vi "test Data Width and Data Loss Error (Integer).vi"(8 "error in (no error)":errorcluster, 11 "TestCase in":refnum<class "BCD.lvclass">) -> (0 "error out":errorcluster, 3 "TestCase out":refnum<class "BCD.lvclass">)   [LabVIEW 2027, in "BCD.lvclass"]
uses:
  BCD.lvclass
  89223b31-db80-4792-afa8-2a57f7cc7b8f.vi
  a83072f1-e87d-421c-9031-0ad09725bb69.vi
  eb97fcc3-29ee-467e-b675-3d761fb83be5.vi
  24b16479-40f3-4730-80e6-3775a7937614.vi
  Source/Get Bits Per Digit from Base.vi
  C:/Program Files/National Instruments/LabVIEW 2027/vi.lib/addons/_JKI Toolkits/VI Tester/TestCase.llb/TestCase.lvclass
  <vilib>/addons/_JKI Toolkits/VI Tester/TestCase.llb/TestCase.lvclass
panel:
  out "BCD encoded value":bool[](array[boolean])
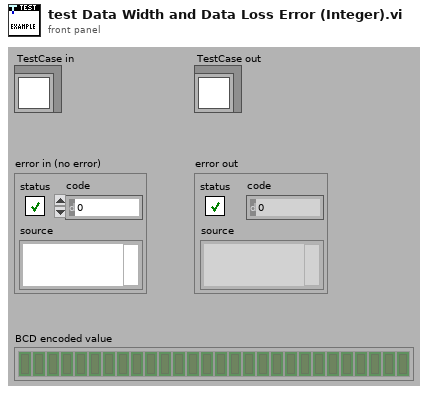
[diagram p1: front panel]
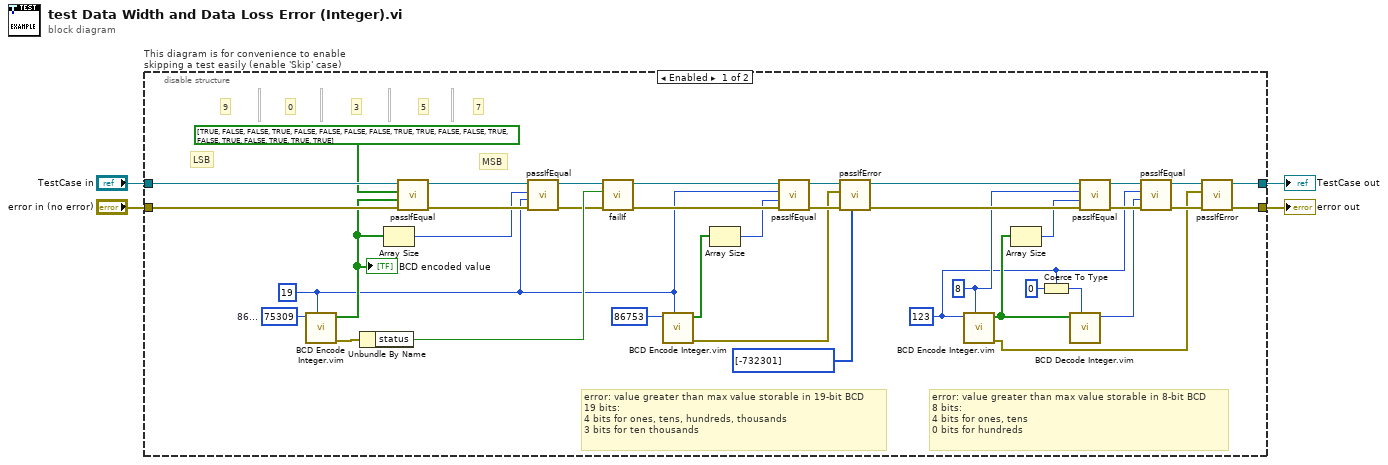
[diagram p0: block diagram]
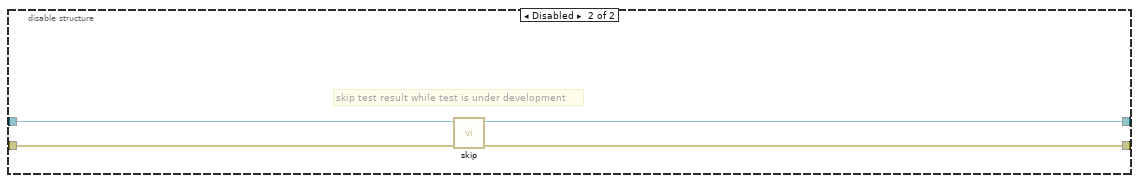
[diagram p2: hidden frame]
diagram:
  n1 = disable-structure "This diagram is for convenience to enable skipping a test easily (enable 'Skip' case)" shown="Enabled" {
    disable-tunnel: "TestCase in" -> [w41 w46]
    disable-tunnel: [w9 w44] -> w1
    disable-tunnel: [w13 w45] -> w3
    disable-tunnel: "error in (no error)" -> [w39 w43]
    frame Enabled {
      w17 = 8 ("data size (bits)")
      w6 = i64 123 ("86...")
      w15 = 19 ("data size (bits)")
      w33 = u32 75309  # 86...
      # "error: value greater than max value storable in 8-bit BCD\n8 bits:\n4 bits for ones, tens\n0 bits for hundreds"
      # "error: value greater than max value storable in 19-bit BCD\n19 bits: \n4 bits for ones, tens, hundreds, thousands\n3 bits for ten thousands"
      # "MSB"
      # "LSB"
      # "9"
      # "0"
      # "3"
      # "5"
      # "7"
      n2 = call "BCD Encode Integer.vim"("data size (bits)"=w15, "integer"=w33) -> ("error out"=w29:errorcluster, "BCD encoded value"=w35:bool[])  [unwired: 8 in]
      "BCD encoded value" <- w35
      n3 = Unbundle By Name(w29) -> ("status"=w28:bool)
      n4 = Array Size(array=w35) -> (size(s)=w34:i32)
      n5 = call-dynamic "passIfEqual.vi"("error in (no error)"=w39, "y"=w35, "x"=bool[] [TRUE, FALSE, FALSE, TRUE, FALSE, FALSE, FALSE, FALSE, TRUE, TRUE, FALSE, FALSE, TRUE, FALSE, TRUE, FALSE, TRUE, TRUE, TRUE] ("BCD encoded value"), "TestCase in"=w41) -> ("error out"=w40:errorcluster, "TestCase out"=w42:refnum<class "BCD.lvclass">)  [unwired: 6 in]
      n6 = call-dynamic "passIfEqual.vi"("error in (no error)"=w40, "y"=w15, "x"=w34, "TestCase in"=w42) -> ("error out"=w26:errorcluster, "TestCase out"=w27:refnum<class "BCD.lvclass">)  [unwired: 6 in]
      n7 = call-dynamic "failIf.vi"("error in (no error)"=w26, "fail"=w28, "TestCase in"=w27) -> ("error out"=w24:errorcluster, "TestCase out"=w25:refnum<class "BCD.lvclass">)  [unwired: 7 in]
      n8 = call "BCD Encode Integer.vim"("data size (bits)"=w15, "integer"=86753 ("86...")) -> ("error out"=w30:errorcluster, "BCD encoded value"=w31:bool[])  [unwired: 8 in]
      n9 = Array Size(array=w31) -> (size(s)=w14:i32)
      n10 = call-dynamic "passIfEqual.vi"("error in (no error)"=w24, "y"=w14, "x"=w15, "TestCase in"=w25) -> ("error out"=w37:errorcluster, "TestCase out"=w38:refnum<class "BCD.lvclass">)  [unwired: 6 in]
      n11 = call-dynamic "passIfError.vi"("passing error codes (default = any error code)"=i32[] [-732301], "error in (no error)"=w37, "error"=w30, "TestCase in"=w38) -> ("error out"=w21:errorcluster, "TestCase out"=w19:refnum<class "BCD.lvclass">)  [unwired: 6 in]
      n12 = call "BCD Encode Integer.vim"("data size (bits)"=w17, "integer"=w6) -> ("error out"=w10:errorcluster, "BCD encoded value"=w20:bool[])  [unwired: 8 in]
      n13 = Array Size(array=w20) -> (size(s)=w16:i32)
      n14 = Coerce To Type(0:0, 1:w6) -> (2:w7:i64)
      n15 = call "BCD Decode Integer.vim"("expected value and type"=w7, "BCD encoded value"=w20) -> ("integer"=w18:i64)  [unwired: 9 in]
      n16 = call-dynamic "passIfEqual.vi"("error in (no error)"=w21, "y"=w16, "x"=w17, "TestCase in"=w19) -> ("error out"=w23:errorcluster, "TestCase out"=w22:refnum<class "BCD.lvclass">)  [unwired: 6 in]
      n17 = call-dynamic "passIfEqual.vi"("error in (no error)"=w23, "y"=w18, "x"=w6, "TestCase in"=w22) -> ("error out"=w11:errorcluster, "TestCase out"=w12:refnum<class "BCD.lvclass">)  [unwired: 6 in]
      n18 = call-dynamic "passIfError.vi"("error in (no error)"=w11, "error"=w10, "TestCase in"=w12) -> ("error out"=w13:errorcluster, "TestCase out"=w9:refnum<class "BCD.lvclass">)  [unwired: 7 in]
    }
    frame Disabled {
      # "skip test result while test is under development"
      n19 = call <vilib>:"skip.vi"("error in (no error)"=w43, "TestCase in"=w46) -> ("error out"=w45:errorcluster, "TestCase out"=w44:refnum<class "BCD.lvclass">)  [unwired: 8 in]
    }
  }
  "error out" <- w3
  "TestCase out" <- w1
